vi "ReadData.vi"(8 "errin":errorcluster caption="entrée d'erreur (pas d'erreur)", 11 "visain":refnum<visa-resource-name>) -> (0 "errout":errorcluster caption="sortie d'erreur", 1 "TResult":string, 2 "VResult":string, 3 "visaout":refnum<visa-resource-name>)   [LabVIEW 2020]
doc: "Lit le package de data venant du arduino"
uses:
  <vilib>/Instr/_visa.llb/VISA Configure Serial Port (Instr).vi
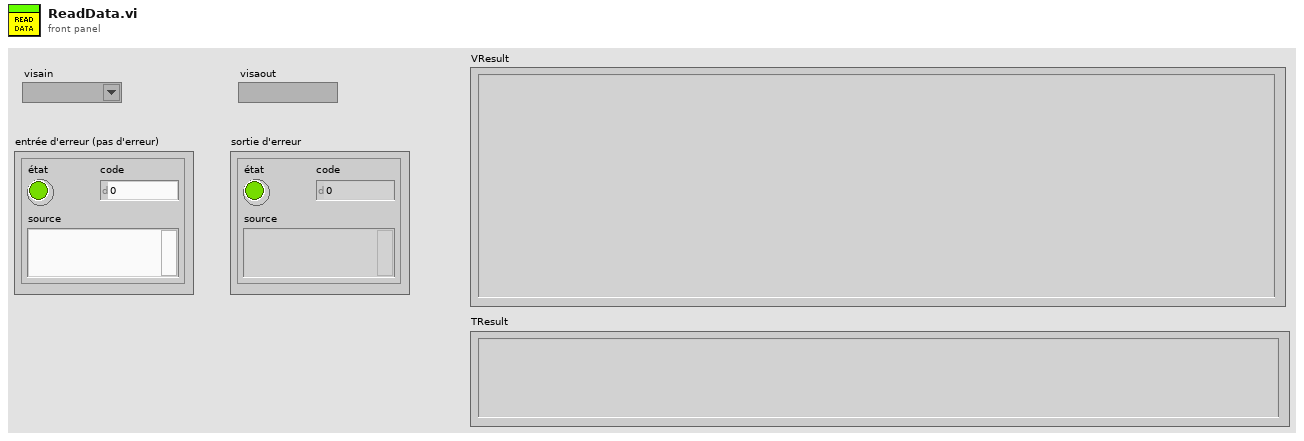
[diagram p1: front panel]
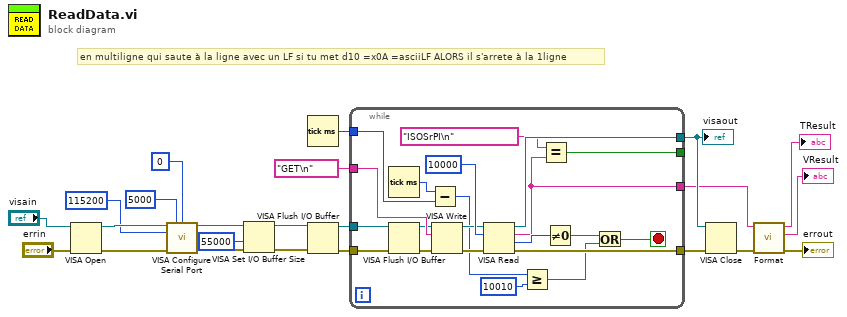
[diagram p0: block diagram]
diagram:
  # "en multiligne qui saute à la ligne avec un LF si tu met d10 =x0A =asciiLF ALORS il s'arrete à la 1ligne"
  n1 = VISA Open(error in (no error)="errin", VISA resource name="visain") -> (VISA resource name=w18:refnum<visa-resource-name>, error out=w19:errorcluster)  [unwired: 3 in]
  n2 = call-poly "VISA Configure Serial Port"("VISA resource name"=w18, "timeout (10sec)"=u32 5000, "termination char\n(0xA = '\\n' = LF)"=u8 0 ("termination char\n(0xA = '\\n' = LF)"), "baud rate (9600)"=u32 115200, "error in (no error)"=w19) -> ("VISA resource name out"=w7:refnum<visa-resource-name>, "error out"=w9:errorcluster)  [unwired: 9 in]
  n3 = VISA Set I/O Buffer Size(VISA resource name=w7, size (4096)=u32 55000 ("taille (4096)"), error in (no error)=w9) -> (VISA resource name out=w6:refnum<visa-resource-name>, error out=w8:errorcluster)  [unwired: 1 in]
  n4 = Tick Count (ms)() -> (millisecond timer value=w15:u32)
  n5 = VISA Flush I/O Buffer(VISA resource name=w6, error in (no error)=w8) -> (VISA resource name out=w13:refnum<visa-resource-name>, error out=w14:errorcluster)  [unwired: 1 in]
  n6 = while {
    tunnel: [w44] -> w10
    tunnel: w14 -> [w36]
    tunnel: "GET\n" ("buffer d'écriture") -> [w41]
    tunnel: w13 -> [w37]
    tunnel: [w39] -> w11
    tunnel: [w32] -> _
    tunnel: w15 -> [w30]
    tunnel: [w24] -> w3
    stop <- w25 stop-if-true
    n7 = Tick Count (ms)() -> (millisecond timer value=w31:u32)
    n8 = VISA Flush I/O Buffer(VISA resource name=w37, error in (no error)=w36) -> (VISA resource name out=w34:refnum<visa-resource-name>, error out=w35:errorcluster)  [unwired: 1 in]
    n9 = Subtract(x=w31, y=w30) -> (x-y=w29:u32)
    n10 = VISA Write(VISA resource name=w34, write buffer=w41, error in (no error)=w35) -> (VISA resource name out=w38:refnum<visa-resource-name>, error out=w40:errorcluster)  [unwired: 1 out]
    n11 = VISA Read(VISA resource name=w38, byte count=u32 10000 ("nombre d'octets"), error in (no error)=w40) -> (VISA resource name out=w39:refnum<visa-resource-name>, read buffer=w24:string, return count=w42:u32, error out=w44:errorcluster)
    n12 = Greater Or Equal? ("Supérieur ou égal ?")(x=w29, y=u32 10010) -> (x >= y?=w27:bool)
    n13 = Equal? ("Égaux ?")(x="ISOSrPI\n", y=w24) -> (x = y?=w32:bool)
    n14 = Not Equal To 0?(x=w42) -> (x != 0?=w26:bool)
    n15 = Or(x=w26, y=w27) -> (x .or. y?=w25:bool)
  }
  "visaout" <- w11
  n16 = VISA Close(VISA resource name=w11, error in (no error)=w10) -> (error out=w20:errorcluster)
  n17 = call "Format.vi"("errin1"=w20, "read buffer en entrée"=w3) -> ("errout"=→"errout":errorcluster, "VResult"=→"VResult":string, "TResult"=→"TResult":string)  [unwired: 7 in]
